vi "String.vi"() -> ()   [LabVIEW 2010]
panel:
  out "Numeric 2":dbl
  out "String 5":string
  out "String 4":string
  out "String 3":string
  out "String 2":string
  out "String":string
  out "Numeric":dbl
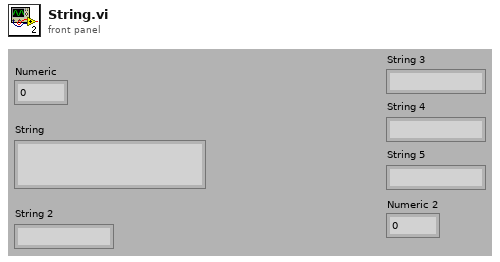
[diagram p1: front panel]
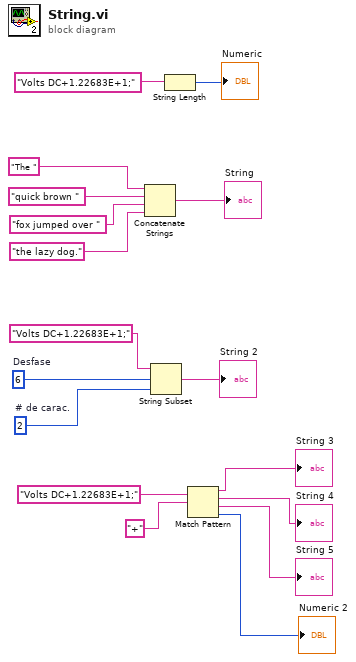
[diagram p0: block diagram]
diagram:
  w9 = 2  # # de carac.
  w10 = 6  # Desfase
  n1 = Concatenate Strings("The ", "quick brown ", "fox jumped over ", "the lazy dog.") -> (→"String":string)
  n2 = String Subset(string="Volts DC+1.22683E+1;", offset (0)=w10, length (rest)=w9) -> (substring=→"String 2":string)
  n3 = String Length(string="Volts DC+1.22683E+1;") -> (length=→"Numeric":i32)
  n4 = Match Pattern(string="Volts DC+1.22683E+1;", regular expression="+") -> (before substring=→"String 3":string, match substring=→"String 4":string, after substring=→"String 5":string, offset past match=→"Numeric 2":i32)  [unwired: 1 in]
